vi "dds_init.vi"(8 "error in":errorcluster, 10 "DDS board initialization parameters":T2={"Bypass PLL"=FALSE, "PLL Range"=TRUE, "Update Clock"=FALSE, "Triangle "=FALSE, "SDO Active"=FALSE, "LSB First"=FALSE, "OSK Int"=FALSE, "Output Shaped Keying Enable"=TRUE, "Bypass Sinc"=FALSE, "Digital Part"=TRUE, "OutPut DAC"=TRUE, "Control DAC"=FALSE, "Comparator"=FALSE, "Modus"=0, "Multiplier Value"=15} {"Modus" scale=0.0..4.0}, 11 "OSK select":bool=TRUE) -> (0 "error out":errorcluster, 3 "constants out":T1)   [LabVIEW 2010]
uses:
  DDS_board_init_cluster.ctl
  FPGA_constants_cluster.ctl
  <vilib>/eio/EIONode/EIONode.xnode
  <vilib>/rvi/eio/nirviEIOImplementation/nirviEIOImplementation.xnode
  <vilib>/rvi/eio/common/nirviEmuClasses.ctl
  <vilib>/rvi/eio/nirviErrorMerge/nirviErrorMerge.xnode
  <vilib>/rvi/eio/common/nirviEmuTemplateMethod_errors.vi
panel:
  # "FSK"
  # "Ramped"
  # "FSK"
  # "Chirp Modus"
  # "Unramped"
  # "BPSK"
  # "Single Tone"
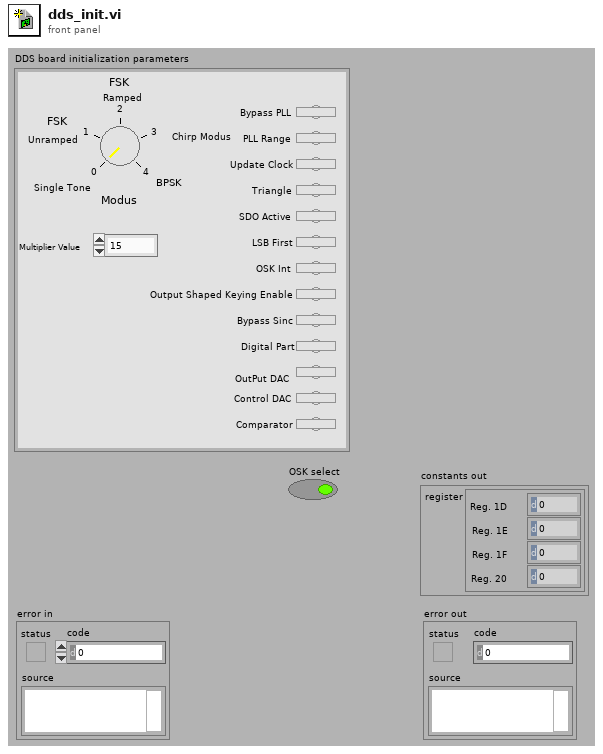
[diagram p1: front panel]
types:
  T1 = typedef "FPGA_constants_cluster.ctl" = cluster{"register":cluster{"Reg. 1D":u8, "Reg. 1E":u8, "Reg. 1F":u8, "Reg. 20":u8}}
  T2 = typedef "DDS_board_init_cluster.ctl" = cluster{"Bypass PLL":bool, "PLL Range":bool, "Update Clock":bool, "Triangle ":bool, "SDO Active":bool, "LSB First":bool, "OSK Int":bool, "Output Shaped Keying Enable":bool, "Bypass Sinc":bool, "Digital Part":bool, "OutPut DAC":bool, "Control DAC":bool, "Comparator":bool, "Modus":u8, "Multiplier Value":u8}
  T3 = typedef "nirviEmuClasses.ctl" = enum16{"IO Read", "IO Write", "Method", "Property Read", "Property Write"}
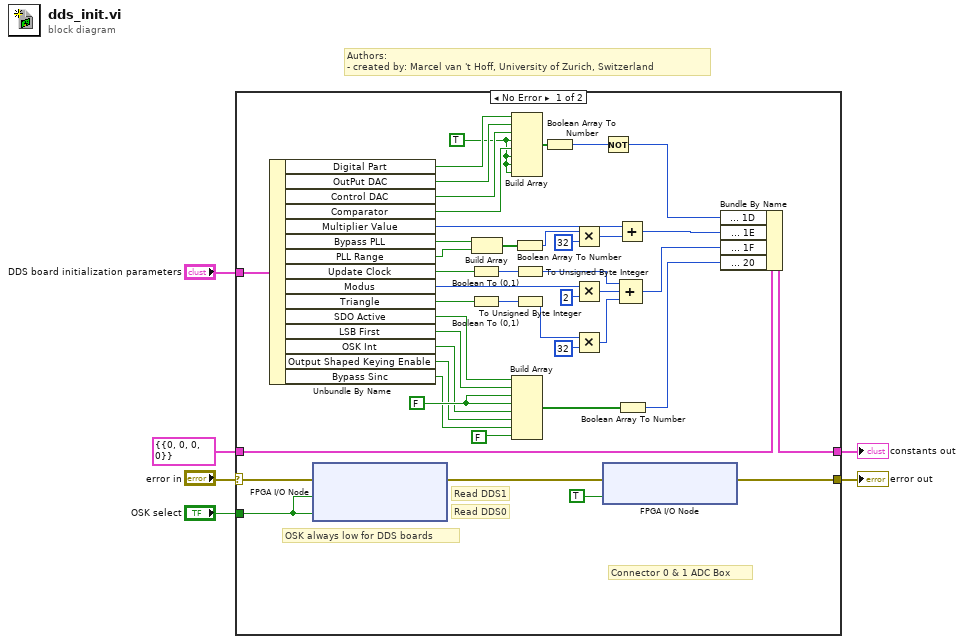
[diagram p0: block diagram]
diagram:
  # "Authors: \n- created by: Marcel van 't Hoff, University of Zurich, Switzerland"
  n1 = case shown="No Error" "error in" {
    selector: "error in" -> [w11 _]
    tunnel: "DDS board initialization parameters" -> [w51 _]
    tunnel: T1 {"register"={"Reg. 1D"=0, "Reg. 1E"=0, "Reg. 1F"=0, "Reg. 20"=0}} ("constants in") -> [w13 _]
    tunnel: [w12 _] -> w4
    tunnel: [w8 _] -> w2
    tunnel: "OSK select" -> [w7 _]
    frame No Error {
      w29 = FALSE
      w30 = TRUE
      # "Read DDS0"
      # "Read DDS1"
      # "Connector 0 & 1 ADC Box"
      # "OSK always low for DDS boards"
      n2 = Unbundle By Name(w51) -> ("Digital Part"=w34:bool, "OutPut DAC"=w33:bool, "Control DAC"=w32:bool, "Comparator"=w31:bool, "Multiplier Value"=w28:u8, "Bypass PLL"=w27:bool, "PLL Range"=w26:bool, "Update Clock"=w21:bool, "Modus"=w20:u8, "Triangle"=w19:bool, "SDO Active"=w18:bool, "LSB First"=w17:bool, "OSK Int"=w16:bool, "Output Shaped Keying Enable"=w15:bool, "Bypass Sinc"=w14:bool)
      n3 = xnode "FPGA I/O Node"("error in"=w11, "Connector3/DIO32"=w7, "Connector3/DIO33"=w7) -> ("error out"=w9:errorcluster)  [unwired: 2 in, 2 out]
      n4 = Boolean To (0,1)(Boolean=w21) -> (0, 1=w44:i16)
      n5 = Boolean To (0,1)(Boolean=w19) -> (0, 1=w38:i16)
      n6 = Build Array(w27, w26) -> (w49:bool[])
      n7 = Build Array(w34, w33, w32, w30, w31, w30, w30, w30) -> (w50:bool[])
      n8 = Build Array(w18, w17, w29, w29, w16, w15, w14, FALSE) -> (w41:bool[])
      n9 = Boolean Array To Number(Boolean array=w49) -> (number=w48:u8)
      n10 = To Unsigned Byte Integer(number=w44) -> (unsigned 8bit integer=w36:u8)
      n11 = To Unsigned Byte Integer(number=w38) -> (unsigned 8bit integer=w37:u8)
      n12 = Boolean Array To Number(Boolean array=w50) -> (number=w39:u8)
      n13 = Multiply(x=w48, y=u8 32) -> (x*y=w46:u8)
      n14 = Multiply(x=w20, y=u8 2) -> (x*y=w35:u8)
      n15 = Multiply(x=w37, y=u8 32) -> (x*y=w42:u8)
      n16 = Not(x=w39) -> (.not. x?=w25:u8)
      n17 = xnode "FPGA I/O Node"("error in"=w9, "Connector0/DIO34"=TRUE ("Connector0/DIO32")) -> ("error out"=w8:errorcluster)  [unwired: 1 in, 1 out]
      n18 = Add(x=w28, y=w46) -> (x+y=w24:u8)
      n19 = Boolean Array To Number(Boolean array=w41) -> (number=w22:u8)
      n20 = Compound Arithmetic op=ADD(w36, w35, w42) -> (w23:u8)
      n21 = Bundle By Name(cluster=w13, "register.Reg. 1D"=w25, "register.Reg. 1E"=w24, "register.Reg. 1F"=w23, "register.Reg. 20"=w22) -> (w12:T1)
    }
    frame Error {
    }
  }
  "constants out" <- w4
  "error out" <- w2
